vi "SaveCycleSweepO.vi"(5 "Area":dbl=1.0, 6 "JunctionName":string, 7 "SideLength":dbl=1.0, 8 "UiDefinition 2":T3, 9 "InfoCluster":T1, 10 "appended array":dbl[][](array[numeric])) -> (0 "error out":errorcluster)   [LabVIEW 2020]
uses:
  UIReferences.ctl
  D:/LabviewDXFViewer/LabviewDXFViewer/bin/Release/LabviewDXFViewer.exe
  LabviewDXFViewer/bin/Release/LabviewDXFViewer.exe
  Keithley_Subs/CapacitanceInfos.ctl
  Keithley_Subs/CapacitanceRecord.ctl
  <vilib>/httpClient/POSTBuffer.vi
  <vilib>/httpClient/LabVIEWHTTPClient.lvlib
panel:
  in  "Cluster 3":T4
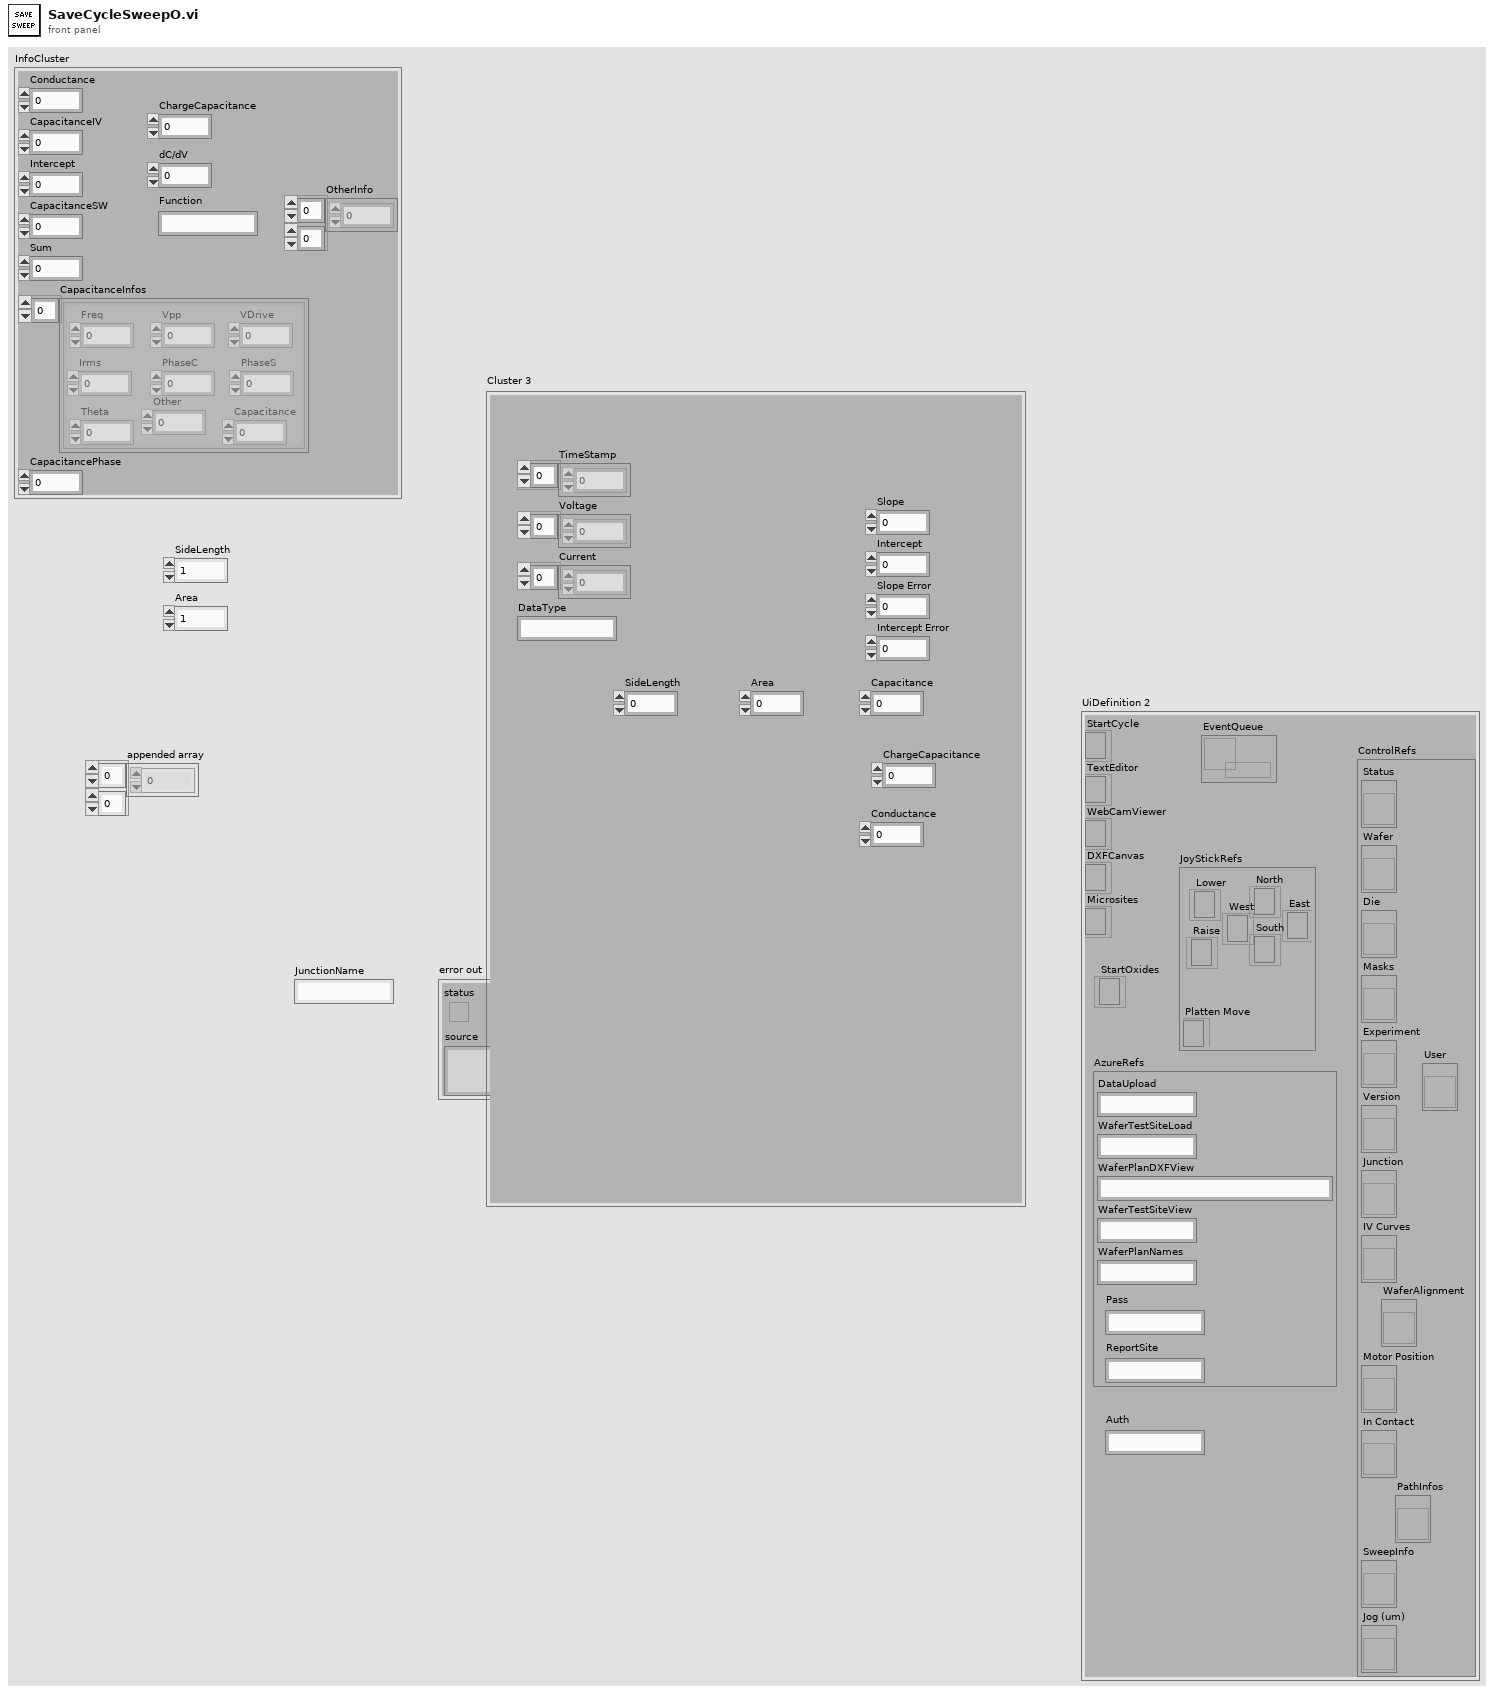
[diagram p1: front panel]
types:
  T1 = typedef "CapacitanceInfos.ctl" = cluster{"Conductance":dbl, "CapacitanceIV":dbl, "Intercept":dbl, "CapacitanceSW":dbl, "Sum":dbl, "CapacitanceInfos":T2[], "CapacitancePhase":dbl, "dC/dV":dbl, "Function":string, "OtherInfo":dbl[][], "ChargeCapacitance":dbl}
  T2 = typedef "CapacitanceRecord.ctl" = cluster{"Freq":dbl, "Vpp":dbl, "PhaseS":dbl, "Irms":dbl, "PhaseC":dbl, "Theta":dbl, "VDrive":dbl, "Capacitance":dbl, "Other":dbl}
  T3 = typedef "UIReferences.ctl" = cluster{"StartCycle":refnum<k24>, "TextEditor":refnum<k24>, "WebCamViewer":refnum<k24>, "DXFCanvas":refnum<k24>, "Microsites":refnum<k24>, "JoyStickRefs":cluster{"North":refnum<k24>, "Lower":refnum<k24>, "Raise":refnum<k24>, "Platten Move":refnum<k24>, "West":refnum<k24>, "East":refnum<k24>, "South":refnum<k24>}, "AzureRefs":cluster{"DataUpload":string, "WaferTestSiteLoad":string, "WaferPlanDXFView":string, "WaferTestSiteView":string, "WaferPlanNames":string, "Pass":string, "ReportSite":string}, "ControlRefs":cluster{"Status":refnum<vi>, "Wafer":refnum<vi>, "Die":refnum<vi>, "Masks":refnum<vi>, "Experiment":refnum<vi>, "Version":refnum<vi>, "Junction":refnum<vi>, "IV Curves":refnum<vi>, "Motor Position":refnum<vi>, "In Contact":refnum<vi>, "SweepInfo":refnum<vi>, "Jog (um)":refnum<vi>, "PathInfos":refnum<vi>, "User":refnum<vi>, "WaferAlignment":refnum<vi>}, "EventQueue":refnum<queue>, "StartOxides":refnum<k24>, "Auth":string}
  T4 = cluster{"Intercept Error":dbl, "Slope Error":dbl, "Intercept":dbl, "Slope":dbl, "DataType":string, "Current":dbl[], "Voltage":dbl[], "TimeStamp":dbl[], "Capacitance":dbl, "Area":dbl, "SideLength":dbl, "ChargeCapacitance":dbl, "Conductance":dbl}
  T5 = cluster{"Die":string, "Wafer":string, "Path":path, "url":string, "Experiment":string, "Version":string, "user":string}
  T6 = typedef "LabVIEWHTTPClient.lvlib/ClientHandle.ctl" = refnum<k1>
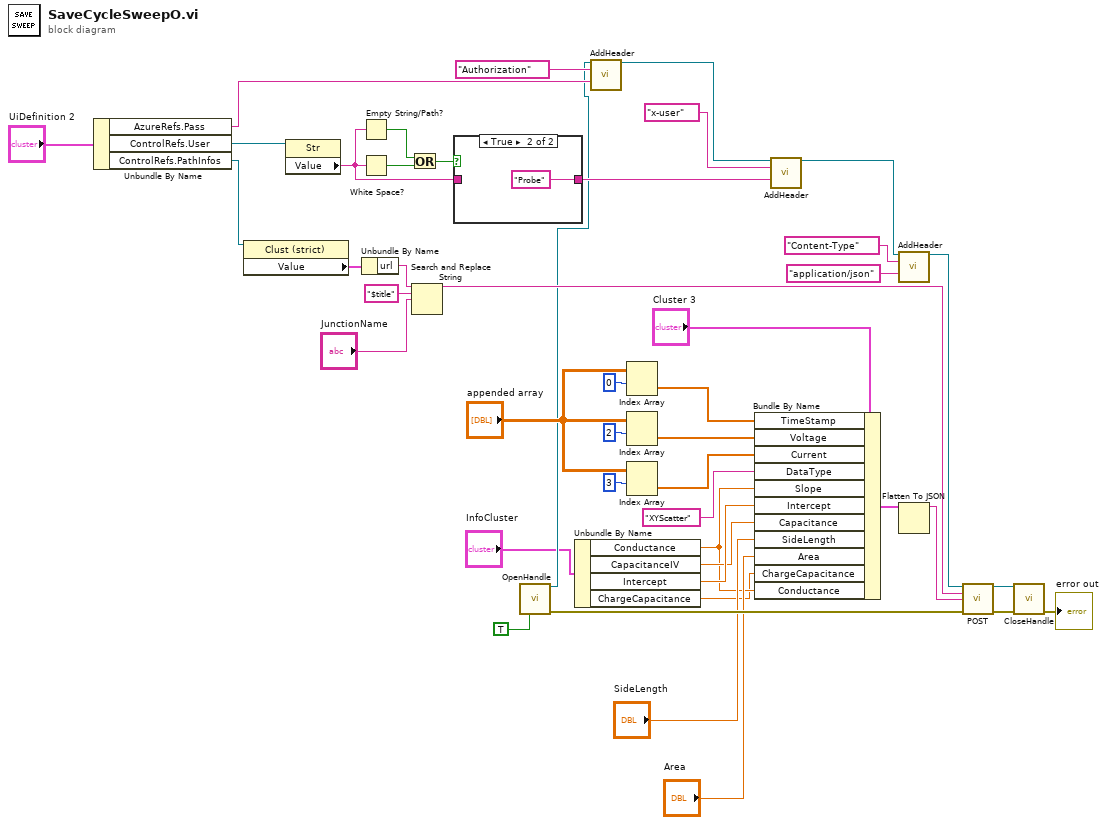
[diagram p0: block diagram]
diagram:
  n1 = Unbundle By Name("UiDefinition 2") -> ("AzureRefs.Pass"=w22:string, "ControlRefs.User"=w20:refnum<vi>, "ControlRefs.PathInfos"=w13:refnum<vi>)
  n2 = property class="Clust (strict)"(reference=w13) -> ("Value"=w12:T5)  [unwired: 1 in, 2 out]
  n3 = property class="Str"(reference=w20) -> ("Value"=w15:string)  [unwired: 1 in, 2 out]
  n4 = Empty String/Path?(string/path=w15) -> (empty?=w16:bool)
  n5 = White Space?(1:w15) -> (0:w19:bool)
  n6 = Unbundle By Name(w12) -> ("url"=w11:string)
  n7 = Or(x=w16, y=w19) -> (x .or. y?=w17:bool)
  n8 = Search and Replace String(input string=w11, search string="$title" ("string"), replace string="JunctionName") -> (result string=w29:string)  [unwired: 5 in, 3 out]
  n9 = case shown="True" w17 {
    tunnel: w15 -> [w46 _]
    tunnel: [w46 "Probe"] -> w18
    frame False {
    }
    frame True {
    }
  }
  n10 = call <vilib>:"OpenHandle.vi"("verify server(true)"=TRUE) -> ("client handle out"=w14:T6, "error out"=w44:errorcluster)  [unwired: 13 in]
  n11 = Unbundle By Name("InfoCluster") -> ("Conductance"=w2:dbl, "CapacitanceIV"=w9:dbl, "Intercept"=w10:dbl, "ChargeCapacitance"=w1:dbl)
  n12 = call <vilib>:"AddHeader.vi"("client handle"=w14, "header"="Authorization", "value"=w22) -> ("client handle out"=w24:T6)  [unwired: 11 in, 1 out]
  n13 = Index Array(array="appended array", index (row)=0) -> (element=w36:dbl[])  [unwired: 1 in]
  n14 = Index Array(array="appended array", index (row)=2) -> (element=w39:dbl[])  [unwired: 1 in]
  n15 = Index Array(array="appended array", index (row)=3) -> (element=w40:dbl[])  [unwired: 1 in]
  n16 = Bundle By Name(cluster="Cluster 3", "TimeStamp"=w36, "Voltage"=w39, "Current"=w40, "DataType"="XYScatter", "Slope"=w2, "Intercept"=w10, "Capacitance"=w9, "SideLength"="SideLength", "Area"="Area", "ChargeCapacitance"=w1, "Conductance"=w2) -> (w43:T4)
  n17 = call <vilib>:"AddHeader.vi"("client handle"=w24, "header"="x-user", "value"=w18) -> ("client handle out"=w4:T6)  [unwired: 11 in, 1 out]
  n18 = call <vilib>:"AddHeader.vi"("client handle"=w4, "header"="Content-Type", "value"="application/json") -> ("client handle out"=w3:T6)  [unwired: 11 in, 1 out]
  n19 = Flatten To JSON(anything=w43) -> (JSON string=w34:string)  [unwired: 2 in, 1 out]
  n20 = call-poly <vilib>:"POST.vi"("client handle"=w3, "url"=w29, "buffer"=w34, "error in (no error)"=w44) -> ("client handle out"=w32:T6, "error out"=w31:errorcluster)  [unwired: 8 in, 2 out]
  n21 = call <vilib>:"CloseHandle.vi"("client handle"=w32, "error in (no error)"=w31) -> ("error out"=→"error out":errorcluster)  [unwired: 13 in]
